vi "Get Tuner Gain.vi"(8 "error in (no error)":errorcluster, 11 "device handle in":T1) -> (0 "error out":errorcluster, 2 "Tuner Gain (dB/10)":i32, 3 "device handle out":T1)   [LabVIEW 2021, in "RTL-SDR.lvlib"]
uses:
  RTL-SDR.lvlib
  usr/lib64/librtlsdr.so.0
  Controls/Device Handle.ctl
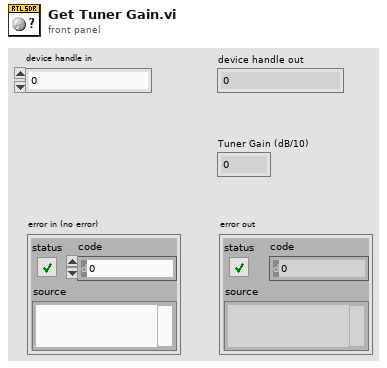
[diagram p1: front panel]
types:
  T1 = typedef "RTL-SDR.lvlib/Device Handle.ctl" = u64
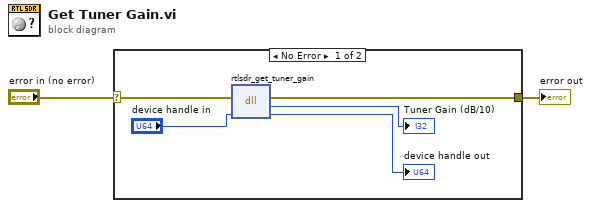
[diagram p0: block diagram]
diagram:
  n1 = case shown="No Error" "error in (no error)" {
    selector: "error in (no error)" -> [w5 w8]
    tunnel: [w4 w8] -> w2
    frame No Error {
      n2 = dll-call lib="usr/lib64/librtlsdr.so.0" fn="rtlsdr_get_tuner_gain"(error in=w5, "dev"="device handle in") -> (error out=w4:errorcluster, "gain"=→"Tuner Gain (dB/10)":i32, "dev"=→"device handle out":u64)  [unwired: 2 in, 1 out]
    }
    frame Error {
    }
  }
  "error out" <- w2
